vi "PosStrikerAnguloAttackerV1.vi"(9 "atacando contra":bool, 10 "IA State":T1={"our_robots"=[], "enemy_robots"=[], "balls"=[], "geometry"={"line_width"=0, "field_length"=0, "field_width"=0, "boundary_width"=0, "referee_width"=0, "goal_width"=0, "goal_depth"=0, "goal_wall_width"=0, "center_circle_radius"=0, "defense_radius"=0, "defense_stretch"=0, "free_kick_from_defense_dist"=0, "penalty_spot_from_field_line_dist"=0, "penalty_line_from_spot_dist"=0}, "IA Judge"={"stage"="", "command"="", "our_goalie_id"=0.0, "enemy_goalie_id"=0.0, "command enum"=enum."Halt", "Time"=enum."Azul"}, "Received Timestamp"=timestamp(0 s since 1904-01-01), "Events"={"Touch"=FALSE, "Ball out"=FALSE, "id touch"=0.0, "Ball out of \nVision"=FALSE, "Ball inside \nGoalie area"=FALSE, "Robot not responding"=FALSE, "Robots responding status"=[1.0, 1.0, 1.0, 1.0, 1.0, 1.0], "Enemy Ball \nPossession"=FALSE, "Pass State"=FALSE, "id end of pass"=0.0, "Kick"=FALSE, "Id ini Possession"=0.0, "Ball Possesion"=FALSE, "Id Possesion"=0.0, "Direct Kick"=FALSE, "2nd Strk Ativo"=FALSE}}) -> (0 "YdoAttacker 2":dbl, 1 "AttackerPositive?":bool, 2 "theta final":dbl, 3 "XdoAttacker 2":dbl)   [LabVIEW 2017]
uses:
  Core/AI Input.ctl
  Core/AI Robot.ctl
  Intel/Functions Enum.ctl
  Intel/AttackerStates.ctl
  Path Planning/RRT/PathDests.ctl
  Path Planning/RRT/PathDest.ctl
  Core/AI Ball.ctl
  Core/Field Size.ctl
  Core/AI Judge.ctl
  Intel/Command Enum.ctl
  Events/Events.ctl
panel:
  in  "valor de theta 3":dbl
  in  "tamanho do intervalo 3":dbl
  in  "inicio do intervalo 3":dbl
  in  "fim do intervalo 3":dbl
  in  "Contador 4":dbl
  in  "Array 3":dbl[](array[numeric])=[0.0, 0.0, 0.0, 0.0, 0.0, 0.0]
  in  "valor de theta 2":dbl
  in  "tamanho do intervalo 2":dbl
  in  "inicio do intervalo 2":dbl
  in  "fim do intervalo 2":dbl
  in  "Contador 3":dbl
  in  "Array 2":dbl[](array[numeric])=[0.0, 0.0, 0.0, 0.0, 0.0, 0.0]
  in  "XdoAttacker":dbl
  in  "YdoAttacker":dbl
  in  "RobôsParaAnalisar":dbl[][](array[numeric])=[[99999.0, 99999.0], [99999.0, 99999.0], [99999.0, 99999.0], [99999.0, 99999.0], [99999.0, 99999.0], [99999.0, 99999.0], [99999.0, 99999.0]]
  in  "Contador":dbl
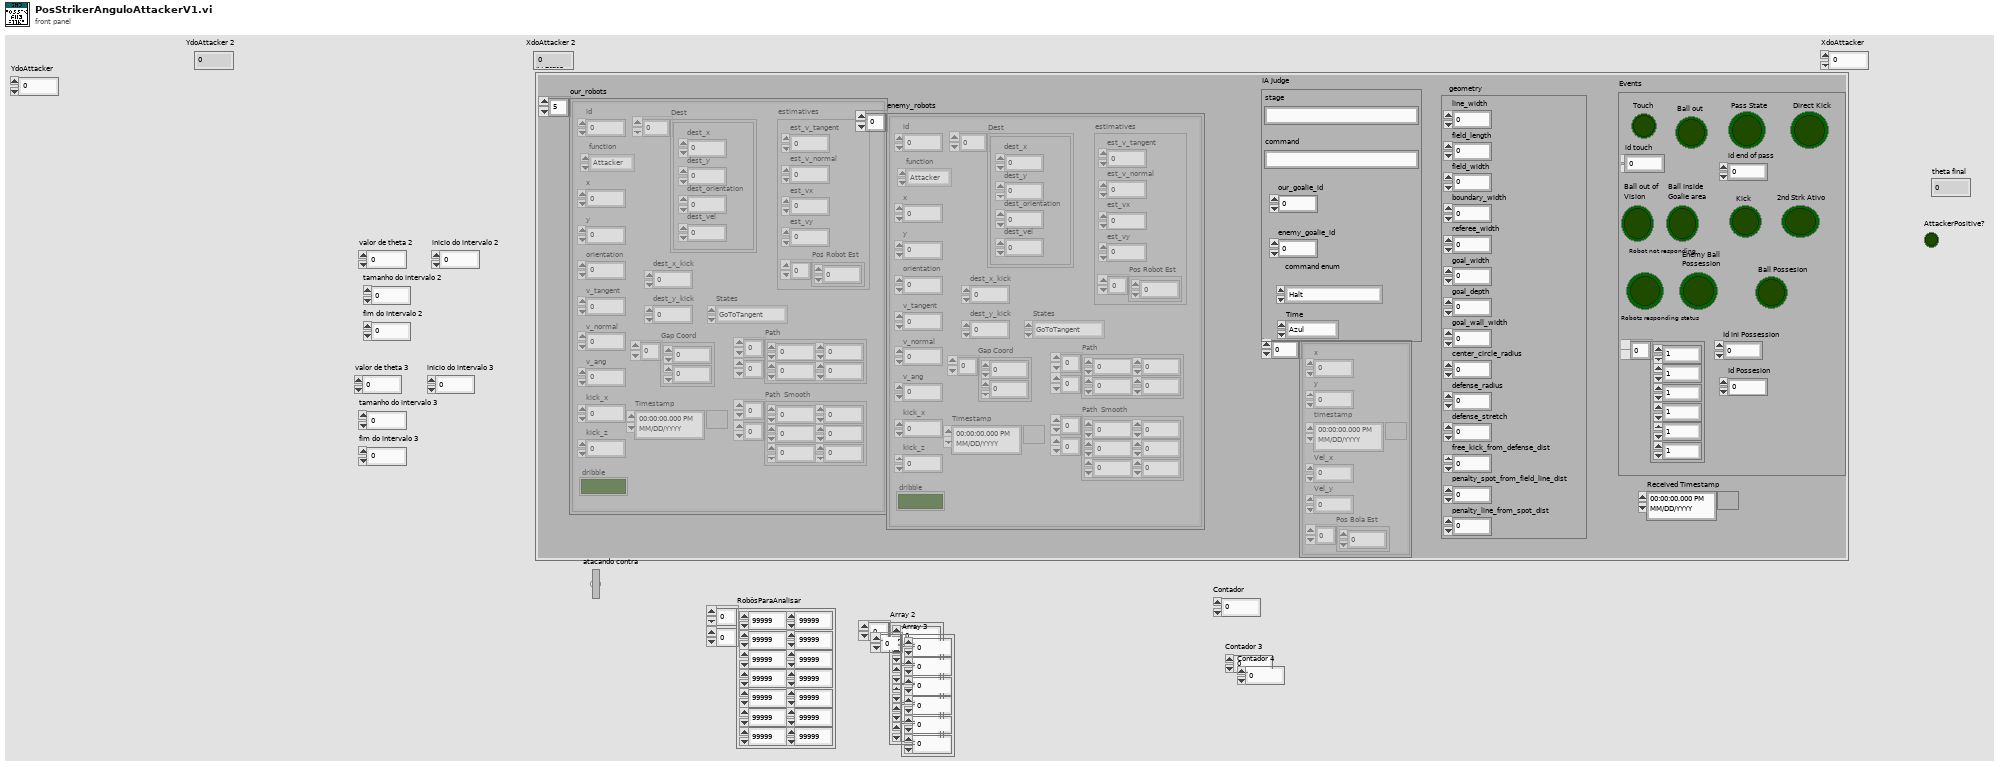
[diagram p1: front panel]
types:
  T1 = typedef "AI Input.ctl" = cluster{"our_robots":T2[], "enemy_robots":T2[], "balls":T7[], "geometry":T8, "IA Judge":T9, "Received Timestamp":timestamp, "Events":T11}
  T2 = typedef "AI Robot.ctl" = cluster{"id":u32, "function":T3, "x":dbl, "y":dbl, "orientation":dbl, "v_tangent":dbl, "v_normal":dbl, "v_ang":dbl, "kick_x":dbl, "kick_z":dbl, "dribble":bool, "Timestamp":timestamp, "estimatives":cluster{"est_v_tangent":dbl, "est_v_normal":dbl, "est_vx":dbl, "est_vy":dbl, "Pos Robot Est":dbl[]}, "dest_x_kick":dbl, "dest_y_kick":dbl, "Gap Coord":dbl[], "States":T4, "Path ":dbl[][], "Path  Smooth":dbl[][], "Dest":T5}
  T3 = typedef "Functions Enum.ctl" = enum16{"2nd Striker", "Attacker", "Goalie", "Defender", "Striker", "Goto 0", "Dummy", "Kicker", "ZigZag 0", "ZigZag 1", "ZigZag 2", "ZigZag 3", "ZigZag 4", "ZigZag 5", "ZigZag 6", "ZigZag 7", "ZigZag 8", ""}
  T4 = typedef "AttackerStates.ctl" = enum16{"Pass", "GoToTangent", "BallGetting", "GoToKick", ""}
  T5 = typedef "PathDests.ctl" = T6[]
  T6 = typedef "PathDest.ctl" = cluster{"dest_x":dbl, "dest_y":dbl, "dest_orientation":dbl, "dest_vel":dbl}
  T7 = typedef "AI Ball.ctl" = cluster{"x":dbl, "y":dbl, "timestamp":timestamp, "Vel_x":dbl, "Vel_y":dbl, "Pos Bola Est":dbl[]}
  T8 = typedef "Field Size.ctl" = cluster{"line_width":u32, "field_length":u32, "field_width":u32, "boundary_width":u32, "referee_width":u32, "goal_width":u32, "goal_depth":u32, "goal_wall_width":u32, "center_circle_radius":u32, "defense_radius":u32, "defense_stretch":u32, "free_kick_from_defense_dist":u32, "penalty_spot_from_field_line_dist":u32, "penalty_line_from_spot_dist":u32}
  T9 = typedef "AI Judge.ctl" = cluster{"stage":string, "command":string, "our_goalie_id":dbl, "enemy_goalie_id":dbl, "command enum":T10, "Time":enum16{"Azul", "Amarelo"}}
  T10 = typedef "Command Enum.ctl" = enum16{"Halt", "Stop", "Force Start", "PKA Normal Start", "Prepare Kickoff Ally", "PKE Normal Start", "Prepare Kickoff Enemy", "Prepare Penalty Ally", "PPA Normal Start", "Prepare Penalty Enemy", "PPE Normal Start", "Direct Free Enemy", "Direct Free Ally", "Indirect Free Enemy", "Indirect Free Ally", "Timeout Enemy", "Timeout Ally", "Goal Enemy", "Goal Ally", "Ball Placement Enemy", "Ball Placement Ally", "Normal Half Time", "Extra Time Break", "Extra Half Time", "None", "Post Game"}
  T11 = typedef "Events.ctl" = cluster{"Touch":bool, "Ball out":bool, "id touch":dbl, "Ball out of \nVision":bool, "Ball inside \nGoalie area":bool, "Robot not responding":bool, "Robots responding status":dbl[], "Enemy Ball \nPossession":bool, "Pass State":bool, "id end of pass":dbl, "Kick":bool, "Id ini Possession":dbl, "Ball Possesion":bool, "Id Possesion":dbl, "Direct Kick":bool, "2nd Strk Ativo":bool}
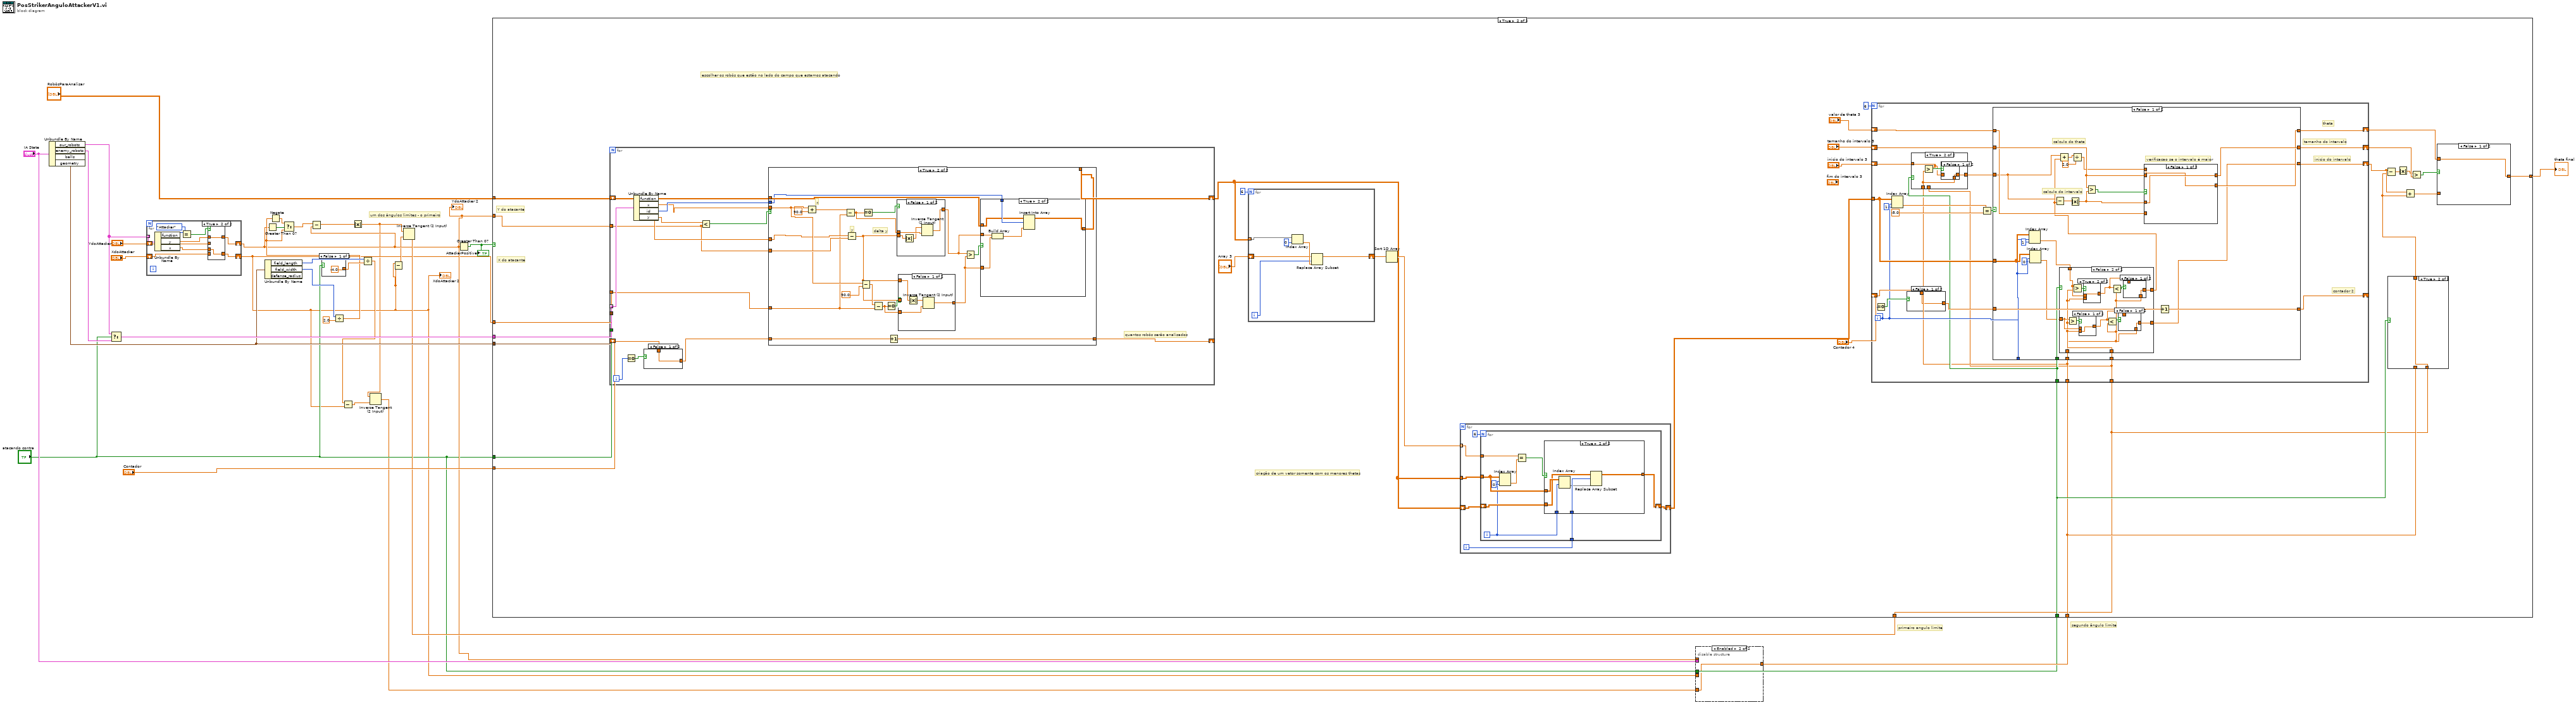
[diagram p0: block diagram]
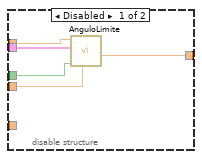
[diagram p2: hidden frame]
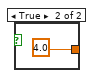
[diagram p3: hidden frame]
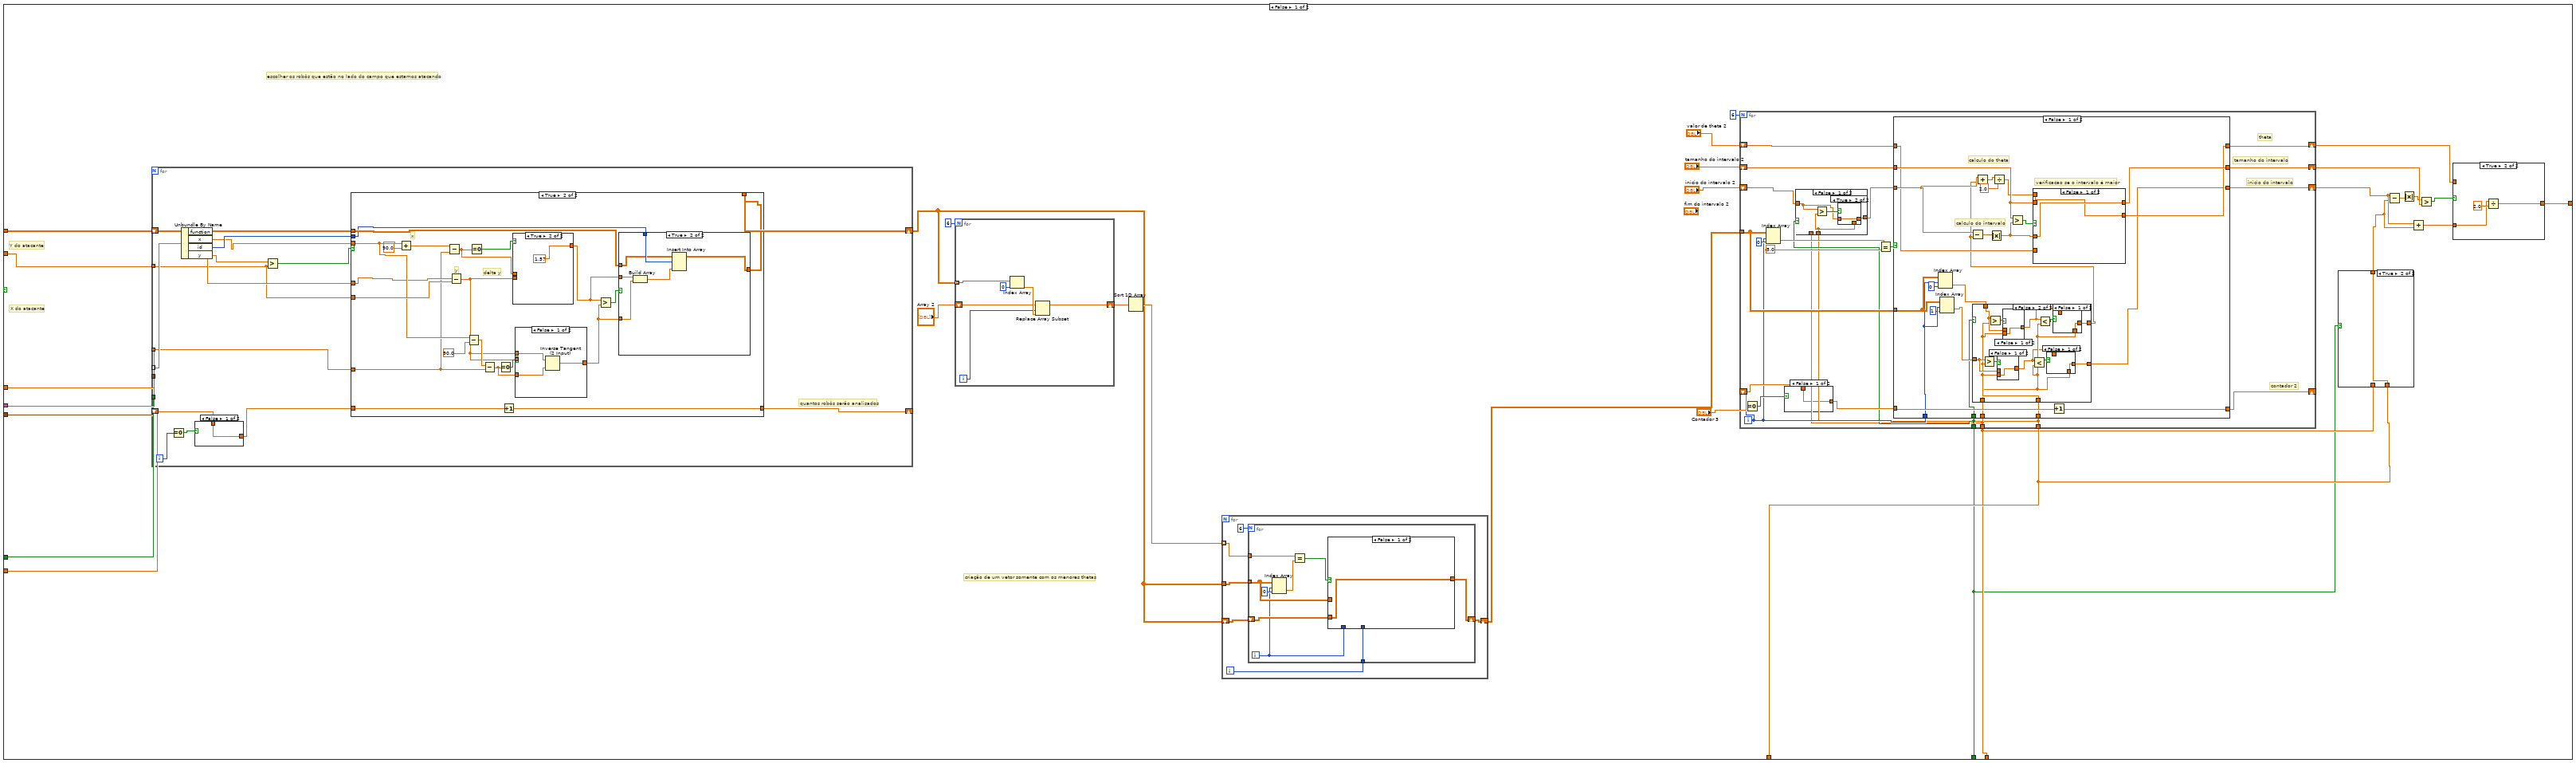
[diagram p4: hidden frame]
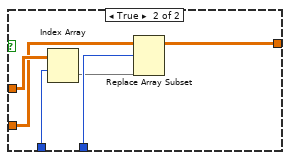
[diagram p7: hidden frame]
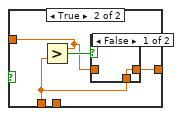
[diagram p9: hidden frame]
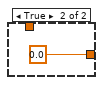
[diagram p11: hidden frame]
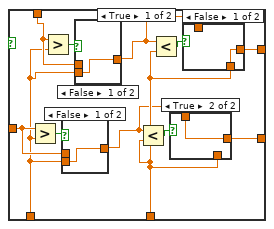
[diagram p12: hidden frame]
diagram:
  # "primeiro angulo limite"
  # "segundo ãngulo limite"
  # "um dos ângulos limites - o primeiro"
  n1 = Unbundle By Name("IA State") -> ("our_robots"=w25:T2[], "enemy_robots"=w30:T2[], "geometry"=w17:T8)  [unwired: 1 out]
  n2 = Select(t=w25, s="atacando contra", f=w30) -> (s? t:f=w29:T2[])
  n3 = for {
    tunnel: w25 -> [w40] mode=indexing
    shift-right: [w35] -> w11
    shift-left: "YdoAttacker" -> [w34]
    shift-right: [w31] -> w4
    shift-left: "XdoAttacker" -> [w32]
    n4 = Unbundle By Name(w40) -> ("function"=w39:T3, "y"=w36:dbl, "x"=w33:dbl)
    n5 = Equal?(x=w39, y=Functions_Enum."Attacker") -> (x = y?=w37:bool)
    n6 = case shown="True" w37 {
      tunnel: w36 -> [_ w44]
      tunnel: [w42 w44] -> w35
      tunnel: w34 -> [w42 _]
      tunnel: w33 -> [_ w43]
      tunnel: w32 -> [w41 _]
      tunnel: [w41 w43] -> w31
      frame False {
      }
      frame True {
      }
    }
  }
  "YdoAttacker 2" <- w11
  "XdoAttacker 2" <- w4
  n7 = Unbundle By Name(w17) -> ("field_length"=w21:u32, "field_width"=w15:u32)  [unwired: 1 out]
  n8 = Greater Than 0?(x=w11) -> (x > 0?=w20:bool)
  n9 = case shown="False" "atacando contra" {
    tunnel: [-4.0 ("y") 4.0 ("y")] -> w18
    frame False {
    }
    frame True {
    }
  }
  n10 = Divide(x=w15, y=2.0) -> (x/y=w14:dbl)
  n11 = Negate(x=w14) -> (-x=w19:dbl)
  n12 = Select(t=w19, s=w20, f=w14) -> (s? t:f=w10:dbl)
  n13 = Subtract(x=w10, y=w11) -> (x-y=w8:dbl)
  n14 = Absolute Value(x=w8) -> (abs(x)=w2:dbl)
  n15 = Divide(x=w21, y=w18) -> (x/y=w5:dbl)
  n16 = Subtract(x=w5, y=w4) -> (x-y=w3:dbl)
  n17 = Inverse Tangent (2 Input)(1:w3, 2:w2) -> (0:w1:dbl)
  n18 = Subtract(x=w4, y=w4) -> (x-y=w9:dbl)
  n19 = Inverse Tangent (2 Input)(1:w9, 2:w2) -> (0:w13:dbl)
  n20 = Greater Than 0?(x=w11) -> (x > 0?=w22:bool)
  "AttackerPositive?" <- w22
  n21 = disable-structure shown="Enabled" {
    disable-tunnel: [w47 w53] -> w12
    disable-tunnel: w11 -> [w52 _]
    disable-tunnel: "IA State" -> [w51 _]
    disable-tunnel: "atacando contra" -> [w50 _]
    disable-tunnel: w4 -> [w49 _]
    disable-tunnel: w1 -> [w48 w53]
    frame Disabled {
      n22 = call "AnguloLimite.vi"("XdoAttacker"=w49, "atacando contra"=w50, "IA State"=w51, "YdoAttacker"=w52) -> ("Angulo Limite"=w47:dbl)  [unwired: 7 in]
    }
    frame Enabled {
    }
  }
  n23 = case shown="True" w22 {
    tunnel: w29 -> [w83 w316]
    tunnel: "atacando contra" -> [w82 w315]
    tunnel: "Contador" -> [w81 w314]
    tunnel: "RobôsParaAnalisar" -> [w80 w313]
    tunnel: w17 -> [w79 w312]
    tunnel: [w65 w298] -> w26
    tunnel: w11 -> [w59 w292]
    tunnel: w4 -> [w58 w291]
    tunnel: w13 -> [w56 w287]
    tunnel: "atacando contra" -> [w54 w290]
    tunnel: w12 -> [w55 w289]
    frame False {
      # "X do atacante"
      # "Y do atacante"
      # "criação de um vetor somente com os menores thetas"
      # "escolher os robôs que estão no lado do campo que estamos atacando"
      n24 = for {
        tunnel: w83 -> [w237] mode=indexing
        tunnel: w82 -> [_]
        shift-right: [w229] -> w69
        shift-left: w80 -> [w236]
        shift-right: [w230] -> _
        shift-left: w81 -> [w232]
        tunnel: w79 -> [_]
        tunnel: w59 -> [w225]
        tunnel: w58 -> [w224]
        i -> [w233]
        # "quantos robôs serão analisados"
        n25 = Equal To 0?(x=w233) -> (x = 0?=w234:bool)
        n26 = Unbundle By Name(w237) -> ("x"=w228:dbl, "id"=w235:u32, "y"=w227:dbl)  [unwired: 1 out]
        n27 = case shown="False" w234 {
          tunnel: w232 -> [w238 _]
          tunnel: [w238 0.0] -> w231
          frame False {
          }
          frame True {
          }
        }
        n28 = Greater?(x=w227, y=w225) -> (0:w226:bool)
        n29 = case shown="True" w226 {
          tunnel: w236 -> [w244 w264]
          tunnel: w235 -> [w243 w263]
          tunnel: w228 -> [_ w254]
          tunnel: w227 -> [_ w253]
          tunnel: w231 -> [w245 w265]
          tunnel: [w245 w266] -> w230
          tunnel: [w240 w262] -> w229
          tunnel: w225 -> [_ w255]
          tunnel: w224 -> [_ w251]
          frame False {
            w242 = -5.0 ("element")
            n30 = Build Array(w242, w242) -> (w241:dbl[])
            n31 = Insert Into Array(array=w244, index (row)=w243, new element=w241) -> (w240:dbl[][])  [unwired: 1 in]
          }
          frame True {
            # "delta y"
            # "y"
            # "x"
            n32 = Add(x=w254, y=90.0) -> (x+y=w252:dbl)
            n33 = Subtract(x=w252, y=w251) -> (x-y=w249:dbl)
            n34 = Subtract(x=w253, y=w255) -> (x-y=w246:dbl)
            n35 = Subtract(x=w254, y=90.0) -> (x-y=w259:dbl)
            n36 = Equal To 0?(x=w249) -> (x = 0?=w250:bool)
            n37 = Subtract(x=w259, y=w251) -> (x-y=w247:dbl)
            n38 = Equal To 0?(x=w247) -> (x = 0?=w248:bool)
            n39 = Increment(x=w265) -> (x+1=w266:dbl)
            n40 = case shown="True" w250 {
              tunnel: [w284 1.57] -> w257
              tunnel: w246 -> [w285 _]
              tunnel: w249 -> [w283 _]
              frame False {
                n41 = Inverse Tangent (2 Input)(1:w283, 2:w285) -> (0:w284:dbl)
              }
              frame True {
              }
            }
            n42 = case shown="False" w248 {
              tunnel: [w269 1.57] -> w256
              tunnel: w246 -> [_ _]
              tunnel: w247 -> [w268 _]
              tunnel: w246 -> [w267 _]
              frame False {
                n43 = Inverse Tangent (2 Input)(1:w268, 2:w267) -> (0:w269:dbl)
              }
              frame True {
              }
            }
            n44 = Greater?(x=w257, y=w256) -> (0:w258:bool)
            n45 = case shown="True" w258 {
              tunnel: w264 -> [w273 w279]
              tunnel: w263 -> [w275 w282]
              tunnel: w257 -> [w272 w280]
              tunnel: w256 -> [w274 w278]
              tunnel: [w271 w277] -> w262
              frame False {
                n46 = Build Array(w274, w272) -> (w276:dbl[])
                n47 = Insert Into Array(array=w273, index (row)=w275, new element=w276) -> (w271:dbl[][])  [unwired: 1 in]
              }
              frame True {
                n48 = Build Array(w280, w278) -> (w281:dbl[])
                n49 = Insert Into Array(array=w279, index (row)=w282, new element=w281) -> (w277:dbl[][])  [unwired: 1 in]
              }
            }
          }
        }
      }
      n50 = for {
        N: 6 -> [_]
        tunnel: w69 -> [w117] mode=indexing
        shift-right: [w112] -> w71
        shift-left: "Array 2" -> [w113]
        i -> [w114]
        n51 = Index Array(array=w117, index=0) -> (element=w115:dbl)
        n52 = Replace Array Subset(array=w113, new element=w115, index=w114) -> (w112:dbl[])
      }
      n53 = Sort 1D Array(array=w71) -> (sorted array=w70:dbl[])
      n54 = for {
        tunnel: w70 -> [w92] mode=indexing
        tunnel: w69 -> [w94]
        shift-right: [w90] -> w68
        shift-left: w69 -> [w93]
        i -> [w91]
        n55 = for {
          N: 6 -> [_]
          tunnel: w94 -> [w100]
          shift-right: [w96] -> w90
          shift-left: w93 -> [w99]
          tunnel: w92 -> [w102]
          tunnel: w91 -> [w97]
          i -> [w98]
          n56 = Index Array(array=w100, index (row)=w98, index (col)=0 ("disabled index (col)")) -> (element=w103:dbl)
          n57 = Equal?(x=w102, y=w103) -> (x = y?=w101:bool)
          n58 = case shown="False" w101 {
            tunnel: w100 -> [_ w111]
            tunnel: w99 -> [w105 w107]
            tunnel: w98 -> [_ w110]
            tunnel: w97 -> [_ w109]
            tunnel: [w105 w106] -> w96
            frame False {
            }
            frame True {
              n59 = Index Array(array=w111, index (row)=w110) -> (element=w108:dbl[])  [unwired: 1 in]
              n60 = Replace Array Subset(array=w107, new element=w108, index (row)=w109) -> (w106:dbl[][])  [unwired: 1 in]
            }
          }
        }
      }
      n61 = for {
        N: 6 -> [_]
        tunnel: w68 -> [w124]
        shift-right: [w132] -> w64
        shift-left: "valor de theta 2" -> [w133]
        shift-right: [w130] -> w67
        shift-left: "tamanho do intervalo 2" -> [w131]
        shift-right: [w129] -> w61
        shift-left: "inicio do intervalo 2" -> [w121]
        shift-right: [w125] -> _
        shift-left: "Contador 3" -> [w127]
        tunnel: w55 -> [w119]
        tunnel: w56 -> [w118]
        tunnel: w54 -> [w122]
        i -> [w123]
        # "contador 2"
        # "inicio do intervalo"
        # "tamanho do intervalo"
        # "theta"
        n62 = Equal To 0?(x=w123) -> (x = 0?=w128:bool)
        n63 = Index Array(array=w124, index (row)=w123, index (col)=0 ("disabled index (col)")) -> (element=w135:dbl)
        n64 = case shown="False" w128 {
          tunnel: w127 -> [w150 _]
          tunnel: [w150 0.0] -> w126
          frame False {
          }
          frame True {
          }
        }
        n65 = case shown="False" w122 {
          tunnel: w119 -> [_ w144]
          tunnel: w121 -> [w140 w145]
          tunnel: [w138 w146] -> w120
          tunnel: w118 -> [w139 _]
          frame False {
            n66 = Greater?(x=w140, y=w139) -> (0:w141:bool)
            n67 = case shown="True" w141 {
              tunnel: [w142 w143] -> w138
              tunnel: w140 -> [_ w143]
              tunnel: w139 -> [w142 _]
              frame False {
              }
              frame True {
              }
            }
          }
          frame True {
            n68 = Greater?(x=w145, y=w144) -> (0:w147:bool)
            n69 = case shown="False" w147 {
              tunnel: [w148 w149] -> w146
              tunnel: w145 -> [_ w149]
              tunnel: w144 -> [w148 _]
              frame False {
              }
              frame True {
              }
            }
          }
        }
        n70 = Equal?(x=w135, y=-5.0) -> (x = y?=w136:bool)
        n71 = case shown="False" w136 {
          tunnel: w133 -> [w159 w223]
          tunnel: [w160 w223] -> w132
          tunnel: w131 -> [w164 w222]
          tunnel: [w163 w222] -> w130
          tunnel: w120 -> [w175 w221]
          tunnel: [w157 w221] -> w129
          tunnel: w126 -> [w173 w220]
          tunnel: [w174 w220] -> w125
          tunnel: w124 -> [w172 _]
          tunnel: w123 -> [w171 _]
          tunnel: w119 -> [w154 _]
          tunnel: w118 -> [w153 _]
          tunnel: w122 -> [w152 _]
          frame False {
            # "calculo do theta"
            # "calculo do intervalo"
            # "verificacao se o intervalo é maior"
            n72 = Index Array(array=w172, index (row)=w171, index (col)=0 ("disabled index (col)")) -> (element=w156:dbl)
            n73 = Index Array(array=w172, index (row)=w171, index (col)=1 ("disabled index (col)")) -> (element=w158:dbl)
            n74 = case shown="False" w152 {
              tunnel: w154 -> [w179 w197]
              tunnel: w156 -> [w186 w206]
              tunnel: w153 -> [w178 w198]
              tunnel: [w184 w204] -> w155
              tunnel: w158 -> [w180 w200]
              tunnel: [w177 w199] -> w157
              frame True {
                n75 = Greater?(x=w180, y=w179) -> (0:w182:bool)
                n76 = Greater?(x=w186, y=w179) -> (0:w187:bool)
                n77 = case shown="False" w182 {
                  tunnel: [w190 w191] -> w176
                  tunnel: w180 -> [_ w191]
                  tunnel: w179 -> [w190 _]
                  frame False {
                  }
                  frame True {
                  }
                }
                n78 = case shown="False" w187 {
                  tunnel: [w194 w195] -> w183
                  tunnel: w186 -> [_ w195]
                  tunnel: w179 -> [w194 _]
                  frame False {
                  }
                  frame True {
                  }
                }
                n79 = Less?(x=w176, y=w178) -> (x < y?=w181:bool)
                n80 = Less?(x=w183, y=w178) -> (x < y?=w185:bool)
                n81 = case shown="True" w181 {
                  tunnel: [w188 w189] -> w177
                  tunnel: w176 -> [_ w189]
                  tunnel: w178 -> [w188 _]
                  frame False {
                  }
                  frame True {
                  }
                }
                n82 = case shown="False" w185 {
                  tunnel: [w192 w193] -> w184
                  tunnel: w183 -> [_ w193]
                  tunnel: w178 -> [w192 _]
                  frame False {
                  }
                  frame True {
                  }
                }
              }
              frame False {
                n83 = Greater?(x=w200, y=w198) -> (0:w202:bool)
                n84 = Greater?(x=w206, y=w198) -> (0:w207:bool)
                n85 = case shown="False" w202 {
                  tunnel: [w210 w211] -> w196
                  tunnel: w200 -> [_ w211]
                  tunnel: w198 -> [w210 _]
                  frame False {
                  }
                  frame True {
                  }
                }
                n86 = case shown="False" w207 {
                  tunnel: [w214 w215] -> w203
                  tunnel: w206 -> [_ w215]
                  tunnel: w198 -> [w214 _]
                  frame False {
                  }
                  frame True {
                  }
                }
                n87 = Less?(x=w196, y=w197) -> (x < y?=w201:bool)
                n88 = Less?(x=w203, y=w197) -> (x < y?=w205:bool)
                n89 = case shown="False" w201 {
                  tunnel: [w208 w209] -> w199
                  tunnel: w196 -> [_ w209]
                  tunnel: w197 -> [w208 _]
                  frame False {
                  }
                  frame True {
                  }
                }
                n90 = case shown="False" w205 {
                  tunnel: [w212 w213] -> w204
                  tunnel: w203 -> [_ w213]
                  tunnel: w197 -> [w212 _]
                  frame False {
                  }
                  frame True {
                  }
                }
              }
            }
            n91 = Subtract(x=w175, y=w155) -> (x-y=w168:dbl)
            n92 = Add(x=w175, y=w155) -> (x+y=w167:dbl)
            n93 = Absolute Value(x=w168) -> (abs(x)=w162:dbl)
            n94 = Divide(x=w167, y=2.0) -> (x/y=w161:dbl)
            n95 = Greater?(x=w164, y=w162) -> (0:w165:bool)
            n96 = case shown="False" w165 {
              tunnel: w164 -> [_ w219]
              tunnel: [w217 w219] -> w163
              tunnel: w162 -> [w217 _]
              tunnel: w159 -> [_ w218]
              tunnel: w161 -> [w216 _]
              tunnel: [w216 w218] -> w160
              frame False {
              }
              frame True {
              }
            }
            n97 = Increment(x=w173) -> (x+1=w174:dbl)
          }
          frame True {
          }
        }
      }
      n98 = case shown="True" w54 {
        tunnel: w55 -> [w84 _]
        tunnel: [w84 w85] -> w57
        tunnel: w56 -> [_ w85]
        frame False {
        }
        frame True {
        }
      }
      n99 = Subtract(x=w61, y=w57) -> (x-y=w63:dbl)
      n100 = Absolute Value(x=w63) -> (abs(x)=w62:dbl)
      n101 = Add(x=w61, y=w57) -> (x+y=w60:dbl)
      n102 = Greater?(x=w62, y=w67) -> (0:w66:bool)
      n103 = case shown="True" w66 {
        tunnel: [w86 w88] -> w65
        tunnel: w64 -> [w86 _]
        tunnel: w60 -> [_ w87]
        frame False {
        }
        frame True {
          n104 = Divide(x=w87, y=2.0) -> (x/y=w88:dbl)
        }
      }
    }
    frame True {
      # "X do atacante"
      # "Y do atacante"
      # "criação de um vetor somente com os menores thetas"
      # "escolher os robôs que estão no lado do campo que estamos atacando"
      n105 = for {
        tunnel: w316 -> [w470] mode=indexing
        tunnel: w315 -> [_]
        shift-right: [w462] -> w302
        shift-left: w313 -> [w469]
        shift-right: [w463] -> _
        shift-left: w314 -> [w465]
        tunnel: w312 -> [_]
        tunnel: w292 -> [w458]
        tunnel: w291 -> [w457]
        i -> [w466]
        # "quantos robôs serão analisados"
        n106 = Equal To 0?(x=w466) -> (x = 0?=w467:bool)
        n107 = Unbundle By Name(w470) -> ("x"=w461:dbl, "id"=w468:u32, "y"=w460:dbl)  [unwired: 1 out]
        n108 = case shown="False" w467 {
          tunnel: w465 -> [w471 _]
          tunnel: [w471 0.0] -> w464
          frame False {
          }
          frame True {
          }
        }
        n109 = Less?(x=w460, y=w458) -> (x < y?=w459:bool)
        n110 = case shown="True" w459 {
          tunnel: w469 -> [w477 w497]
          tunnel: w468 -> [w476 w496]
          tunnel: w461 -> [_ w487]
          tunnel: w460 -> [_ w486]
          tunnel: w464 -> [w478 w498]
          tunnel: [w478 w499] -> w463
          tunnel: [w473 w495] -> w462
          tunnel: w458 -> [_ w488]
          tunnel: w457 -> [_ w484]
          frame False {
            w475 = -5.0 ("element")
            n111 = Build Array(w475, w475) -> (w474:dbl[])
            n112 = Insert Into Array(array=w477, index (row)=w476, new element=w474) -> (w473:dbl[][])  [unwired: 1 in]
          }
          frame True {
            # "delta y"
            # "y"
            # "x"
            n113 = Add(x=w487, y=90.0) -> (x+y=w485:dbl)
            n114 = Subtract(x=w485, y=w484) -> (x-y=w482:dbl)
            n115 = Subtract(x=w486, y=w488) -> (x-y=w479:dbl)
            n116 = Subtract(x=w487, y=90.0) -> (x-y=w492:dbl)
            n117 = Equal To 0?(x=w482) -> (x = 0?=w483:bool)
            n118 = Subtract(x=w492, y=w484) -> (x-y=w480:dbl)
            n119 = Equal To 0?(x=w480) -> (x = 0?=w481:bool)
            n120 = Increment(x=w498) -> (x+1=w499:dbl)
            n121 = case shown="False" w483 {
              tunnel: [w520 1.57] -> w490
              tunnel: w479 -> [w518 _]
              tunnel: w482 -> [w519 _]
              frame False {
                n122 = Absolute Value(x=w518) -> (abs(x)=w517:dbl)
                n123 = Inverse Tangent (2 Input)(1:w519, 2:w517) -> (0:w520:dbl)
              }
              frame True {
              }
            }
            n124 = case shown="False" w481 {
              tunnel: [w503 1.57] -> w489
              tunnel: w479 -> [_ _]
              tunnel: w480 -> [w502 _]
              tunnel: w479 -> [w500 _]
              frame False {
                n125 = Absolute Value(x=w500) -> (abs(x)=w501:dbl)
                n126 = Inverse Tangent (2 Input)(1:w502, 2:w501) -> (0:w503:dbl)
              }
              frame True {
              }
            }
            n127 = Greater?(x=w490, y=w489) -> (0:w491:bool)
            n128 = case shown="True" w491 {
              tunnel: w497 -> [w507 w513]
              tunnel: w496 -> [w509 w516]
              tunnel: w490 -> [w506 w514]
              tunnel: w489 -> [w508 w512]
              tunnel: [w505 w511] -> w495
              frame False {
                n129 = Build Array(w508, w506) -> (w510:dbl[])
                n130 = Insert Into Array(array=w507, index (row)=w509, new element=w510) -> (w505:dbl[][])  [unwired: 1 in]
              }
              frame True {
                n131 = Build Array(w514, w512) -> (w515:dbl[])
                n132 = Insert Into Array(array=w513, index (row)=w516, new element=w515) -> (w511:dbl[][])  [unwired: 1 in]
              }
            }
          }
        }
      }
      n133 = for {
        N: 6 -> [_]
        tunnel: w302 -> [w350] mode=indexing
        shift-right: [w345] -> w304
        shift-left: "Array 3" -> [w346]
        i -> [w347]
        n134 = Index Array(array=w350, index=0) -> (element=w348:dbl)
        n135 = Replace Array Subset(array=w346, new element=w348, index=w347) -> (w345:dbl[])
      }
      n136 = Sort 1D Array(array=w304) -> (sorted array=w303:dbl[])
      n137 = for {
        tunnel: w303 -> [w325] mode=indexing
        tunnel: w302 -> [w327]
        shift-right: [w323] -> w301
        shift-left: w302 -> [w326]
        i -> [w324]
        n138 = for {
          N: 6 -> [_]
          tunnel: w327 -> [w333]
          shift-right: [w329] -> w323
          shift-left: w326 -> [w332]
          tunnel: w325 -> [w335]
          tunnel: w324 -> [w330]
          i -> [w331]
          n139 = Index Array(array=w333, index (row)=w331, index (col)=0 ("disabled index (col)")) -> (element=w336:dbl)
          n140 = Equal?(x=w335, y=w336) -> (x = y?=w334:bool)
          n141 = case shown="True" w334 {
            tunnel: w333 -> [_ w344]
            tunnel: w332 -> [w338 w340]
            tunnel: w331 -> [_ w343]
            tunnel: w330 -> [_ w342]
            tunnel: [w338 w339] -> w329
            frame False {
            }
            frame True {
              n142 = Index Array(array=w344, index (row)=w343) -> (element=w341:dbl[])  [unwired: 1 in]
              n143 = Replace Array Subset(array=w340, new element=w341, index (row)=w342) -> (w339:dbl[][])  [unwired: 1 in]
            }
          }
        }
      }
      n144 = for {
        N: 6 -> [_]
        tunnel: w301 -> [w357]
        shift-right: [w365] -> w297
        shift-left: "valor de theta 3" -> [w366]
        shift-right: [w363] -> w300
        shift-left: "tamanho do intervalo 3" -> [w364]
        shift-right: [w362] -> w294
        shift-left: "inicio do intervalo 3" -> [w353]
        shift-right: [w358] -> _
        shift-left: "Contador 4" -> [w360]
        tunnel: w290 -> [w355]
        tunnel: w289 -> [w354]
        tunnel: w287 -> [w351]
        i -> [w356]
        # "contador 2"
        # "inicio do intervalo"
        # "tamanho do intervalo"
        # "theta"
        n145 = Equal To 0?(x=w356) -> (x = 0?=w361:bool)
        n146 = Index Array(array=w357, index (row)=w356, index (col)=1 ("disabled index (col)")) -> (element=w368:dbl)
        n147 = case shown="False" w361 {
          tunnel: w360 -> [w383 _]
          tunnel: [w383 0.0] -> w359
          frame False {
          }
          frame True {
          }
        }
        n148 = case shown="True" w355 {
          tunnel: w354 -> [_ w377]
          tunnel: w353 -> [w373 w378]
          tunnel: [w371 w379] -> w352
          tunnel: w351 -> [w372 _]
          frame False {
            n149 = Greater?(x=w373, y=w372) -> (0:w374:bool)
            n150 = case shown="True" w374 {
              tunnel: [w375 w376] -> w371
              tunnel: w373 -> [_ w376]
              tunnel: w372 -> [w375 _]
              frame False {
              }
              frame True {
              }
            }
          }
          frame True {
            n151 = Greater?(x=w378, y=w377) -> (0:w380:bool)
            n152 = case shown="False" w380 {
              tunnel: [w381 w382] -> w379
              tunnel: w378 -> [_ w382]
              tunnel: w377 -> [w381 _]
              frame False {
              }
              frame True {
              }
            }
          }
        }
        n153 = Equal?(x=w368, y=-5.0) -> (x = y?=w369:bool)
        n154 = case shown="False" w369 {
          tunnel: w366 -> [w393 w456]
          tunnel: [w394 w456] -> w365
          tunnel: w364 -> [w398 w455]
          tunnel: [w397 w455] -> w363
          tunnel: [w387 w453] -> w362
          tunnel: w359 -> [w407 w454]
          tunnel: [w408 w454] -> w358
          tunnel: w357 -> [w406 _]
          tunnel: w356 -> [w405 _]
          tunnel: w355 -> [w392 _]
          tunnel: w354 -> [w391 _]
          tunnel: w351 -> [w390 _]
          tunnel: w352 -> [w386 w453]
          frame False {
            # "calculo do theta"
            # "calculo do intervalo"
            # "verificacao se o intervalo é maior"
            n155 = Index Array(array=w406, index (row)=w405, index (col)=1 ("disabled index (col)")) -> (element=w385:dbl)
            n156 = Index Array(array=w406, index (row)=w405, index (col)=0 ("disabled index (col)")) -> (element=w388:dbl)
            n157 = case shown="False" w392 {
              tunnel: w391 -> [w412 w430]
              tunnel: w385 -> [w419 w439]
              tunnel: w390 -> [w411 w431]
              tunnel: [w417 w437] -> w389
              tunnel: w388 -> [w413 w433]
              tunnel: [w410 w432] -> w387
              frame True {
                n158 = Greater?(x=w413, y=w412) -> (0:w415:bool)
                n159 = Greater?(x=w419, y=w412) -> (0:w420:bool)
                n160 = case shown="False" w415 {
                  tunnel: [w423 w424] -> w409
                  tunnel: w413 -> [_ w424]
                  tunnel: w412 -> [w423 _]
                  frame False {
                  }
                  frame True {
                  }
                }
                n161 = case shown="False" w420 {
                  tunnel: [w427 w428] -> w416
                  tunnel: w419 -> [_ w428]
                  tunnel: w412 -> [w427 _]
                  frame False {
                  }
                  frame True {
                  }
                }
                n162 = Less?(x=w409, y=w411) -> (x < y?=w414:bool)
                n163 = Less?(x=w416, y=w411) -> (x < y?=w418:bool)
                n164 = case shown="True" w414 {
                  tunnel: [w421 w422] -> w410
                  tunnel: w409 -> [_ w422]
                  tunnel: w411 -> [w421 _]
                  frame False {
                  }
                  frame True {
                  }
                }
                n165 = case shown="True" w418 {
                  tunnel: [w425 w426] -> w417
                  tunnel: w416 -> [_ w426]
                  tunnel: w411 -> [w425 _]
                  frame False {
                  }
                  frame True {
                  }
                }
              }
              frame False {
                n166 = Greater?(x=w433, y=w431) -> (0:w435:bool)
                n167 = Greater?(x=w439, y=w431) -> (0:w440:bool)
                n168 = case shown="False" w435 {
                  tunnel: [w443 w444] -> w429
                  tunnel: w433 -> [_ w444]
                  tunnel: w431 -> [w443 _]
                  frame False {
                  }
                  frame True {
                  }
                }
                n169 = case shown="True" w440 {
                  tunnel: [w447 w448] -> w436
                  tunnel: w439 -> [_ w448]
                  tunnel: w431 -> [w447 _]
                  frame False {
                  }
                  frame True {
                  }
                }
                n170 = Less?(x=w429, y=w430) -> (x < y?=w434:bool)
                n171 = Less?(x=w436, y=w430) -> (x < y?=w438:bool)
                n172 = case shown="False" w434 {
                  tunnel: [w441 w442] -> w432
                  tunnel: w429 -> [_ w442]
                  tunnel: w430 -> [w441 _]
                  frame False {
                  }
                  frame True {
                  }
                }
                n173 = case shown="False" w438 {
                  tunnel: [w445 w446] -> w437
                  tunnel: w436 -> [_ w446]
                  tunnel: w430 -> [w445 _]
                  frame False {
                  }
                  frame True {
                  }
                }
              }
            }
            n174 = Subtract(x=w386, y=w389) -> (x-y=w402:dbl)
            n175 = Add(x=w386, y=w389) -> (x+y=w401:dbl)
            n176 = Absolute Value(x=w402) -> (abs(x)=w396:dbl)
            n177 = Divide(x=w401, y=2.0) -> (x/y=w395:dbl)
            n178 = Greater?(x=w398, y=w396) -> (0:w399:bool)
            n179 = case shown="False" w399 {
              tunnel: w398 -> [_ w452]
              tunnel: [w450 w452] -> w397
              tunnel: w396 -> [w450 _]
              tunnel: w393 -> [_ w451]
              tunnel: w395 -> [w449 _]
              tunnel: [w449 w451] -> w394
              frame False {
              }
              frame True {
              }
            }
            n180 = Increment(x=w407) -> (x+1=w408:dbl)
          }
          frame True {
          }
        }
      }
      n181 = case shown="True" w290 {
        tunnel: w289 -> [w317 _]
        tunnel: [w317 w318] -> w288
        tunnel: w287 -> [_ w318]
        frame False {
        }
        frame True {
        }
      }
      n182 = Subtract(x=w294, y=w288) -> (x-y=w296:dbl)
      n183 = Absolute Value(x=w296) -> (abs(x)=w295:dbl)
      n184 = Add(x=w294, y=w288) -> (x+y=w293:dbl)
      n185 = Greater?(x=w295, y=w300) -> (0:w299:bool)
      n186 = case shown="False" w299 {
        tunnel: [w319 w321] -> w298
        tunnel: w297 -> [w319 _]
        tunnel: w293 -> [_ w320]
        frame False {
        }
        frame True {
          n187 = Divide(x=w320, y=2.0) -> (x/y=w321:dbl)
        }
      }
    }
  }
  "theta final" <- w26
